vi "Start Test.vi"(8 "error in (no error)":errorcluster, 10 "Tests":string[](array[string]), 11 "XML Report in":refnum<class "Report Plugin.lvclass">) -> (0 "error out":errorcluster, 3 "XML Report out":refnum<class "Report Plugin.lvclass">)   [LabVIEW 2020, in "Report Plugin.lvclass"]
uses:
  Report Plugin.lvclass
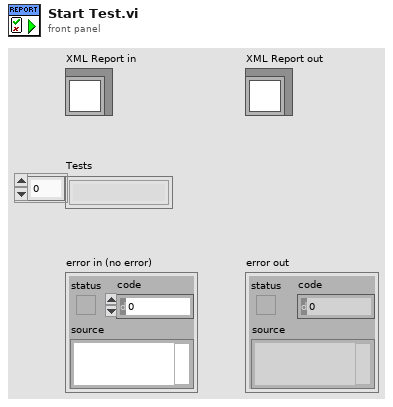
[diagram p1: front panel]
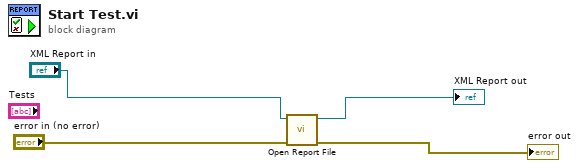
[diagram p0: block diagram]
diagram:
  n1 = call-dynamic "Open Report File.vi"("error in (no error)"="error in (no error)", "Report In"="XML Report in") -> ("error out"=→"error out":errorcluster, "Report Out"=→"XML Report out":refnum<class "Report Plugin.lvclass">)  [unwired: 8 in]
